vi "Custom Aggregation (Deviation).vi"(0 "Urms-under [V]":dbl[](array[numeric]), 1 "reset? (F)":bool, 5 "Urms-over [V]":dbl[](array[numeric]), 7 "aggregation settings":T1={"interval"=1, "interval unit"=enum."Runs", "synchronization of intervals"=enum."Not synchronized", "algorithm"=enum."RMS"}, 9 "system info in":refnum<class "EP System Info.lvclass">, 11 "error in (no error)":errorcluster, 12 "data timestamp":timestamp) -> (4 "Uunder [%]":dbl[](array[numeric]), 6 "Uover [%]":dbl[](array[numeric]), 10 "system info out":refnum<class "EP System Info.lvclass">, 13 "aggregated data valid?":bool, 14 "aggregated data timestamp":timestamp, 15 "error out":errorcluster)   [LabVIEW 2014, in "NI_EP_Power Quality.lvlib"]
doc: "Calculates the aggregated minimum, maximum, and averaged or RMS value of an input signal for a specified aggregation interval, according to Class S in IEC 61000-4-30:2008. There is no overlap between aggregation intervals. This VI automatically restarts accumulation at the beginning of the next time interval after the previous interval expires. You must manually select the polymorphic instance you want to use.\n\nThis VI supports measuring single-line and multiple-line systems except the DBL instance. Use the DBL instance to measure one channel on one line at one time."
uses:
  <vilib>/addons/Electrical Power/PQ/NI_EP_Power Quality.lvlib
  <vilib>/addons/Electrical Power/PQ/Common/Controls/ep_Aggregation Settings.ctl
  <vilib>/addons/Electrical Power/PQ/Common/Classes/System Info/EP System Info.lvclass
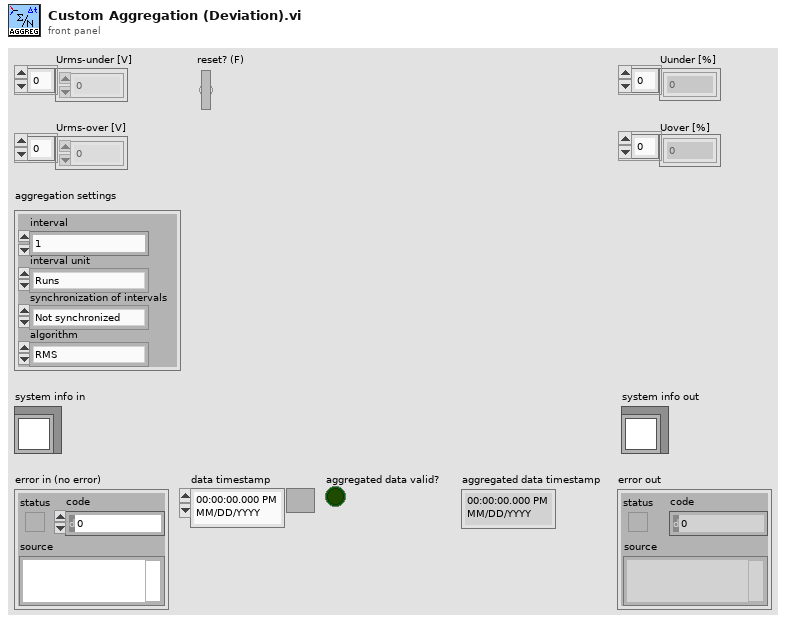
[diagram p1: front panel]
types:
  T1 = typedef "NI_EP_Power Quality.lvlib/ep_Aggregation Settings.ctl" = cluster{"interval":u32, "interval unit":enum16{"Runs", "Seconds", "Minutes", "Hours", "Days", "Weeks"}, "synchronization of intervals":enum16{"Not synchronized", "Interval rounded"}, "algorithm":enum16{"Average", "RMS"}}
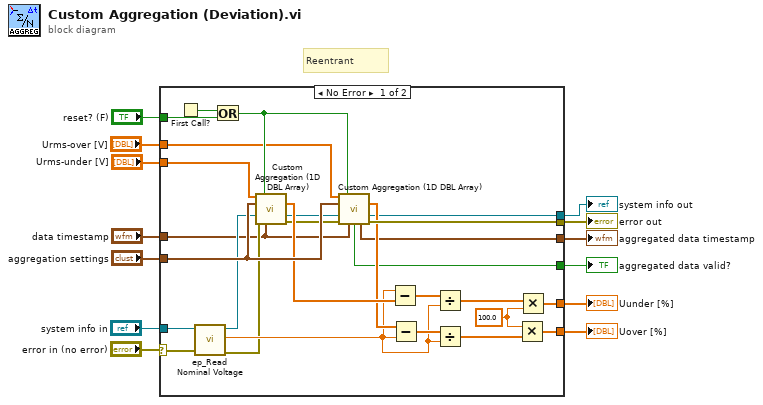
[diagram p0: block diagram]
diagram:
  # "Reentrant"
  n1 = case shown="No Error" "error in (no error)" {
    selector: "error in (no error)" -> [w21 w41]
    tunnel: "reset? (F)" -> [w37 _]
    tunnel: [w40 w41] -> w12
    tunnel: [w16 _] -> w11
    tunnel: "data timestamp" -> [w14 _]
    tunnel: "aggregation settings" -> [w39 _]
    tunnel: [w20 _] -> w8
    tunnel: "Urms-under [V]" -> [w35 _]
    tunnel: "Urms-over [V]" -> [w34 _]
    tunnel: [w29 _] -> w4
    tunnel: [w28 _] -> w3
    tunnel: "system info in" -> [w26 _]
    tunnel: [w17 _] -> w1
    frame No Error {
      w30 = 100.0
      n2 = First Call?() -> (First Call?: T/F=w38:bool)
      n3 = call <vilib>:"ep_Read Nominal Voltage.vi"("error in (no error)"=w21, "system info in"=w26) -> ("error out"=w15:errorcluster, "nominal voltage [V]"=w22:dbl, "system info out"=w18:refnum<class "EP System Info.lvclass">)  [unwired: 7 in]
      n4 = Or(x=w38, y=w37) -> (x .or. y?=w36:bool)
      n5 = call <vilib>:"Custom Aggregation (1D DBL Array).vi"("data in"=w35, "reset? (F)"=w36, "aggregation settings"=w39, "system info in"=w18, "error in (no error)"=w15, "data timestamp"=w14) -> ("aggregated averaged/RMS values"=w33:dbl[], "system info out"=w19:refnum<class "EP System Info.lvclass">, "error out"=w27:errorcluster)  [unwired: 3 in, 4 out]
      n6 = call <vilib>:"Custom Aggregation (1D DBL Array).vi"("data in"=w34, "reset? (F)"=w36, "aggregation settings"=w39, "system info in"=w19, "error in (no error)"=w27, "data timestamp"=w14) -> ("aggregated averaged/RMS values"=w32:dbl[], "system info out"=w17:refnum<class "EP System Info.lvclass">, "aggregated data valid?"=w16:bool, "aggregated data timestamp"=w20:timestamp, "error out"=w40:errorcluster)  [unwired: 3 in, 2 out]
      n7 = Subtract(x=w22, y=w33) -> (x-y=w31:dbl[])
      n8 = Subtract(x=w32, y=w22) -> (x-y=w24:dbl[])
      n9 = Divide(x=w31, y=w22) -> (x/y=w25:dbl[])
      n10 = Divide(x=w24, y=w22) -> (x/y=w23:dbl[])
      n11 = Multiply(x=w30, y=w23) -> (x*y=w28:dbl[])
      n12 = Multiply(x=w25, y=w30) -> (x*y=w29:dbl[])
    }
    frame Error {
    }
  }
  "error out" <- w12
  "aggregated data valid?" <- w11
  "aggregated data timestamp" <- w8
  "Uunder [%]" <- w4
  "Uover [%]" <- w3
  "system info out" <- w1
